vi "initialize.vi"(0 "HGF_Rendezvous":refnum<class "HGF_Rendezvous.lvclass">, 3 "initializationData":variant, 5 "error in (no error)":errorcluster, 7 "binaryString":string, 8 "I8 Array":i8[](array[numeric]), 9 "prependSize? (T)":bool, 11 "byteOrder (0:big-endian, network order)":T1(ring)) -> (14 "dup HGF_Rendezvous":refnum<class "HGF_Rendezvous.lvclass">, 17 "found?":bool, 19 "error out":errorcluster)   [LabVIEW 2014, in "HGF_BaseClasses.lvlib" / "HGF_Rendezvous.lvclass"]
doc: "This is a dynamic dispatch VI to be implemented by child classes to initialize their attributes.\n\n<B>Recommendation:</B> Use Variant for initialization data."
uses:
  HGF_Rendezvous.lvclass
  HGF_InternalEvent/HGF_InternalEvent.lvclass
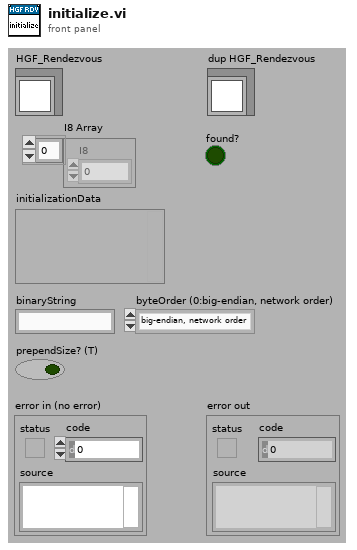
[diagram p1: front panel]
types:
  T1 = enum16{"big-endian, network order", "native, host order", "little-endian"}
  T2 = typedef "Rendezvous RefNum" = refnum<k1>
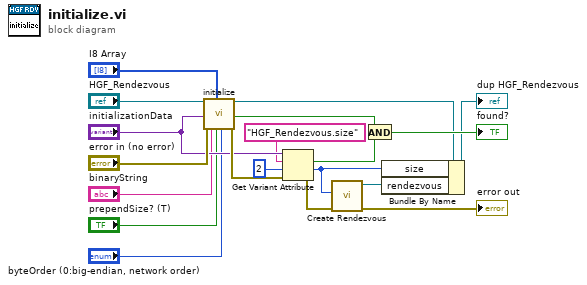
[diagram p0: block diagram]
diagram:
  n1 = call-parent "initialize.vi"("HGF_Timing"="HGF_Rendezvous", "initializationData"="initializationData", "error in (no error)"="error in (no error)", "binaryString"="binaryString", "I8 Array"="I8 Array", "prependSize? (T)"="prependSize? (T)", "byteOrder (0:big-endian, network order)"="byteOrder (0:big-endian, network order)") -> ("dup HGF_Timing"=w8:refnum<class "HGF_Rendezvous.lvclass">, "found?"=w11:bool, "error out"=w16:errorcluster)  [unwired: 1 in, 9 out]
  n2 = Get Variant Attribute(Variant="initializationData", name="HGF_Rendezvous.size", default value (empty Variant)=2, error in=w16) -> (found=w12:bool, value=w7:i32, error out=w9:errorcluster)  [unwired: 1 out]
  n3 = call <vilib>:"Create Rendezvous.vi"("error in (no error)"=w9, "size (2)"=w7) -> ("error out"=→"error out":errorcluster, "rendezvous"=w5:T2)  [unwired: 4 out]
  n4 = And(x=w11, y=w12) -> (x .and. y?=→"found?":bool)
  n5 = Bundle By Name(cluster=w8, "size"=w7, "rendezvous"=w5) -> (→"dup HGF_Rendezvous":refnum<class "HGF_Rendezvous.lvclass">)
